vi "Read Command to Execute.vi"(8 "error in (no error)":errorcluster, 11 "User Defined Write in":refnum<class "User Defined Write.lvclass">) -> (0 "error out":errorcluster, 2 "Command to Execute":string, 3 "User Defined Write out":refnum<class "User Defined Write.lvclass">)   [LabVIEW 2023, in "HAF.lvlib" / "User Defined Write.lvclass"]
doc: "Returns the command to run."
uses:
  User Defined Write.lvclass
  User Defined Write.lvclass/User Defined Write.ctl
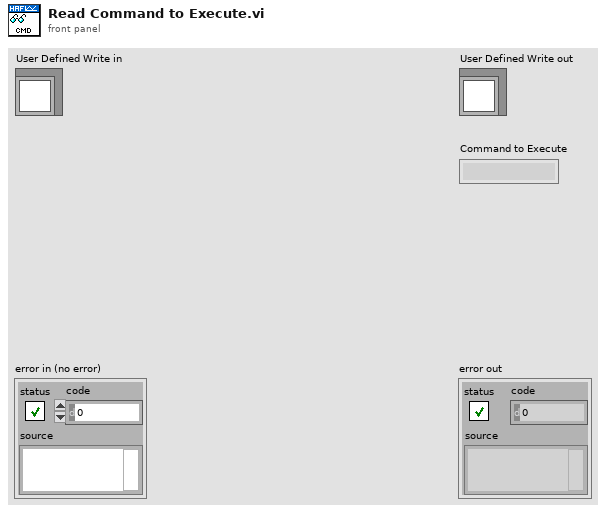
[diagram p1: front panel]
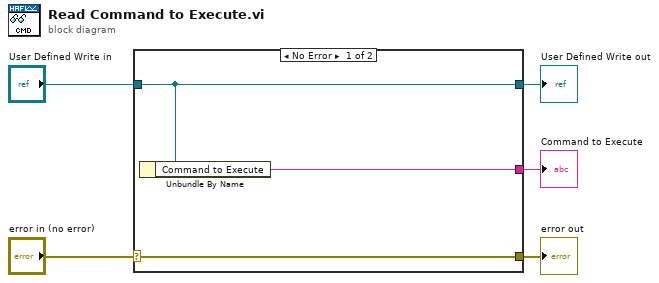
[diagram p0: block diagram]
diagram:
  n1 = case shown="No Error" "error in (no error)" {
    selector: "error in (no error)" -> [w8 w9]
    tunnel: [w8 w9] -> w4
    tunnel: [w7 w10] -> w2
    tunnel: "User Defined Write in" -> [w7 w10]
    tunnel: [w6 _] -> w1
    frame No Error {
      n2 = Unbundle By Name(w7) -> ("Command to Execute"=w6:string)
    }
    frame Error {
    }
  }
  "error out" <- w4
  "User Defined Write out" <- w2
  "Command to Execute" <- w1
